vi "TP Editor-Save.vi"(5 "File Name":string, 8 "path":path) -> (0 "error out":errorcluster, 1 "Cancel":bool, 2 "File Name 2":string)   [LabVIEW 2018]
uses:
  Global.vi
panel:
  in  "Cancel":bool
  in  "OK":bool
  in  "Program list":i32(listbox)
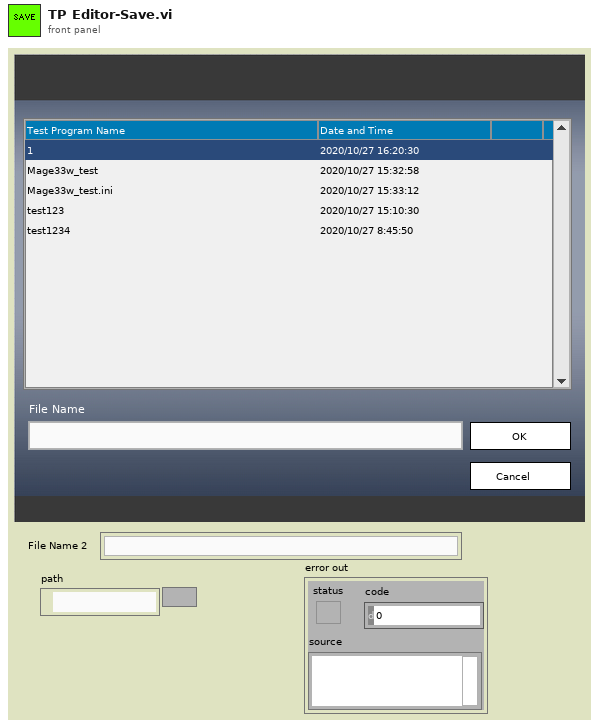
[diagram p1: front panel]
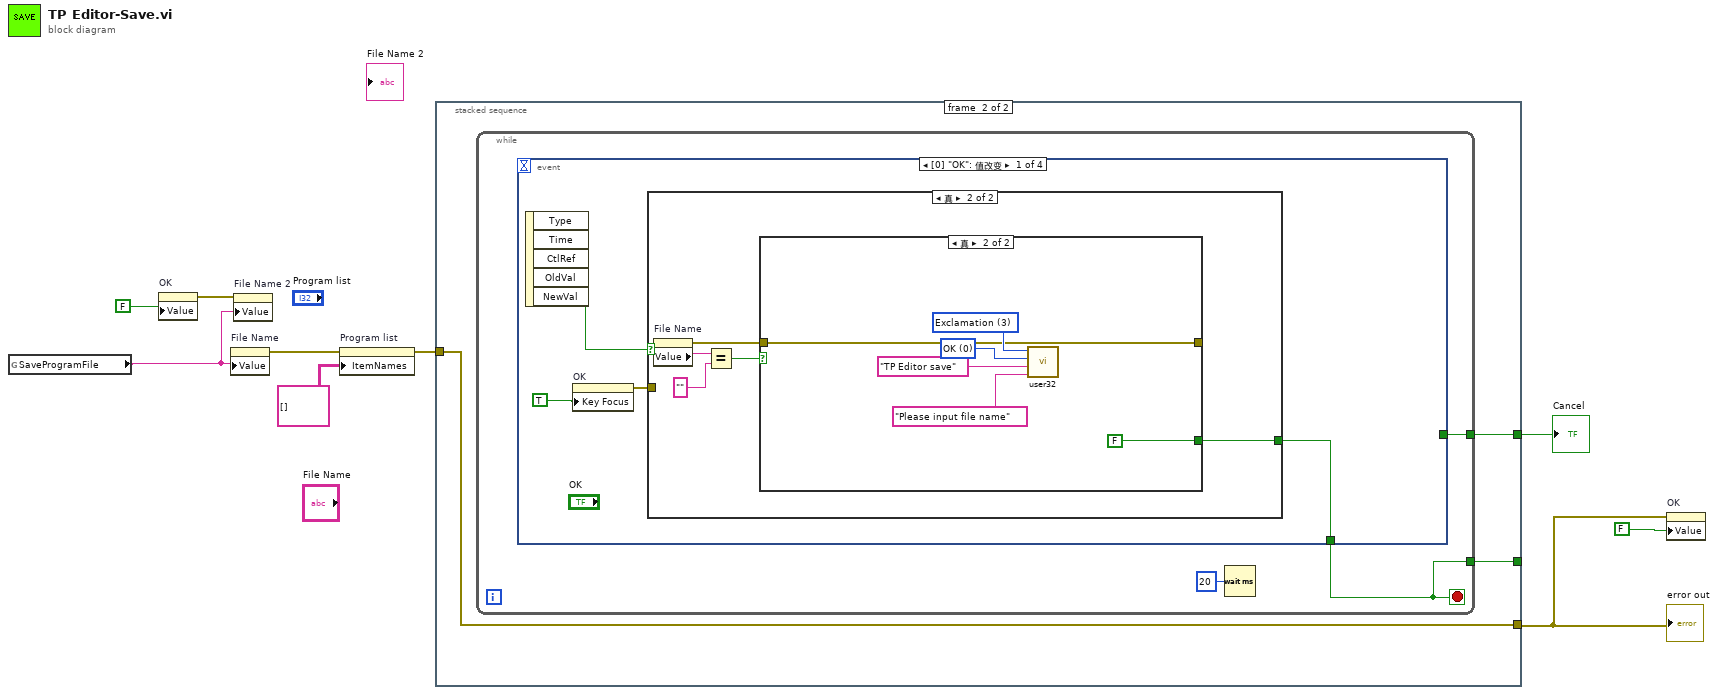
[diagram p0: block diagram]
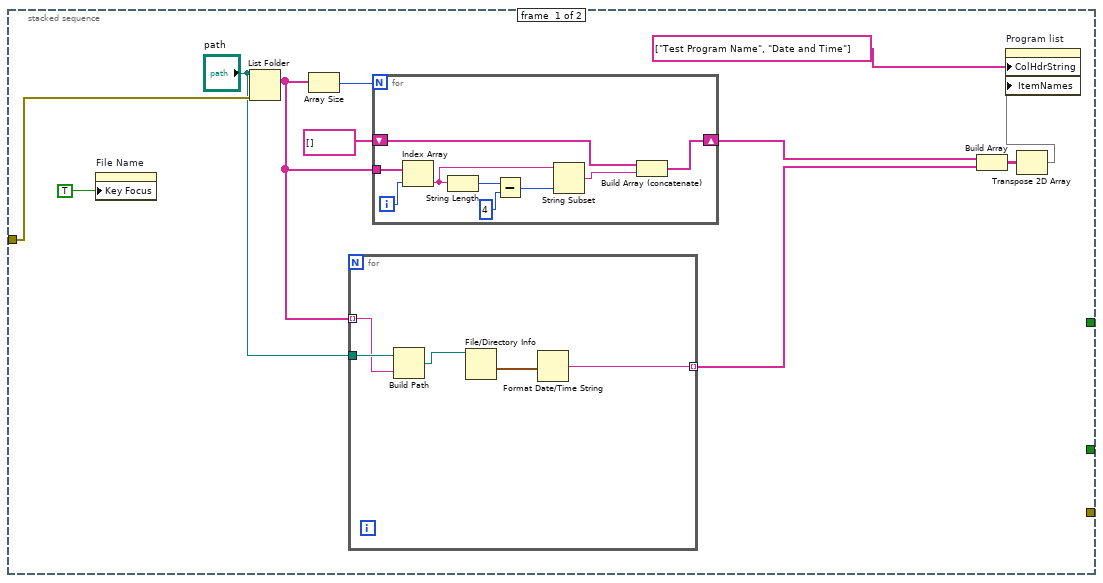
[diagram p2: hidden frame]
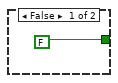
[diagram p3: hidden frame]
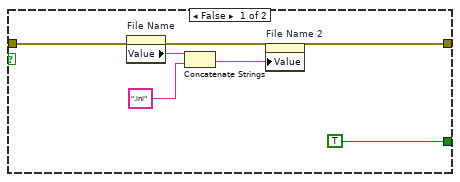
[diagram p4: hidden frame]
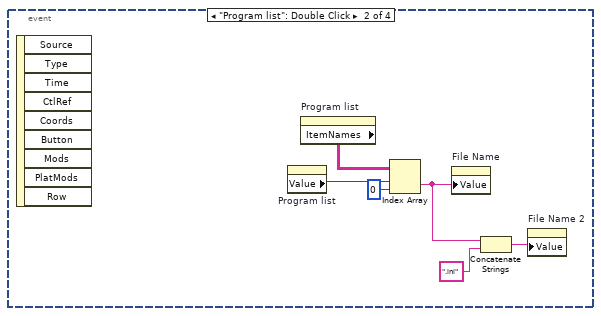
[diagram p5: hidden frame]
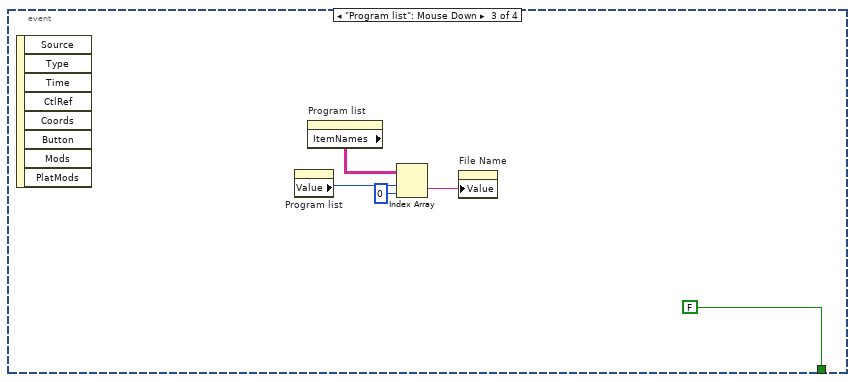
[diagram p6: hidden frame]
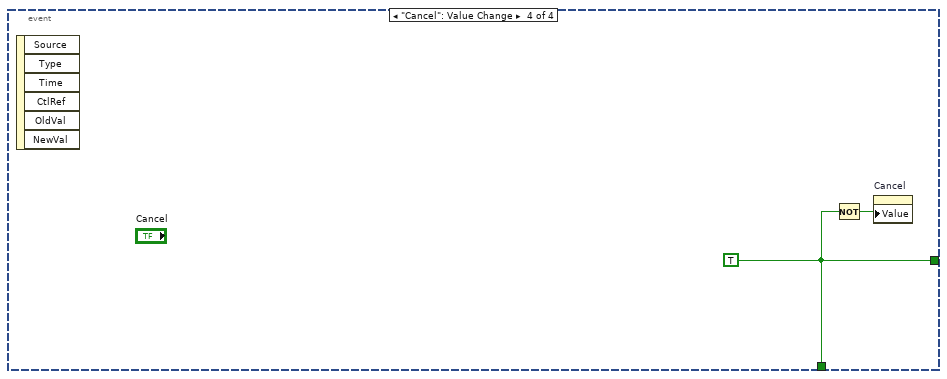
[diagram p7: hidden frame]
diagram:
  n1 = global read "Global.vi" "SaveProgramFile"() -> (w1:string)
  n2 = property on="OK" class="Bool (严格)"("Value"=FALSE) -> (error out=w3:errorcluster)  [unwired: 2 in, 1 out]
  n3 = property on="File Name" class="Str"("Value"=w1) -> (error out=w7:errorcluster)  [unwired: 2 in, 1 out]
  n4 = property on="File Name 2" class="Str"(error in=w3, "Value"=w1) -> ()  [unwired: 1 in, 2 out]
  n5 = property on="Program list" class="MCListbox (严格)"(error in=w7, "ItemNames"=string[][] []) -> (error out=w8:errorcluster)  [unwired: 1 in, 1 out]
  n6 = stacked-sequence {
    tunnel: [_ w37] -> _
    tunnel: w8 -> [w16 w36]
    tunnel: [_ w36] -> w4
    tunnel: [_ w35] -> w6
    frame #0 {
      n7 = property on="File Name" class="Str"("Key Focus"=TRUE) -> ()  [unwired: 2 in, 2 out]
      n8 = List Folder(path="path", error in=w16) -> (filenames=w15:string[])  [unwired: 5 out]
      n9 = Array Size(array=w15) -> (size(s)=w19:i32)
      n10 = for {
        tunnel: w15 -> [w24] mode=indexing
        tunnel: "path" -> [w25]
        tunnel: [w21] -> w11 mode=indexing
        n11 = Build Path(base path=w25, name or relative path=w24) -> (appended path=w23:path)
        n12 = File/Directory Info(path=w23) -> (last mod=w22:timestamp)  [unwired: 1 in, 6 out]
        n13 = Format Date/Time String(seconds (now)=w22) -> (date/time string=w21:string)  [unwired: 2 out]
      }
      n14 = for {
        N: w19 -> [_]
        tunnel: w15 -> [w34]
        shift-right: [w27] -> w10
        shift-left: string[] [] -> [w26]
        i -> [w33]
        n15 = Index Array(array=w34, index=w33) -> (element=w30:string)
        n16 = String Length(string=w30) -> (length=w32:i32)
        n17 = Subtract(x=w32, y=4) -> (x-y=w29:i32)
        n18 = String Subset(string=w30, length (rest)=w29) -> (substring=w28:string)  [unwired: 1 out]
        n19 = Build Array (concatenate)(w26, w28) -> (w27:string[])
      }
      n20 = Build Array(w10, w11) -> (w14:string[][])
      n21 = Transpose 2D Array(2D array=w14) -> (transposed array=w13:string[][])
      n22 = property on="Program list" class="MCListbox (严格)"("ColHdrString"=string[] ["Test Program Name", "Date and Time"] ("Column Header Strings[]"), "ItemNames"=w13) -> ()  [unwired: 2 in, 2 out]
    }
    frame #1 {
      n23 = while {
        tunnel: [w39] -> w37
        tunnel: [w38] -> w35
        stop <- w39 stop-if-true
        n24 = event shown="[0] \"OK\": 值改变" {
          selector: _ -> [_ _ _ _]
          dyn-events: _ -> [_ _ _ _]
          timeout: _ -> [_ _ _ _]
          tunnel: [w44 _ FALSE w73] -> w39
          tunnel: [_ _ _ w73] -> w38
          event "OK": Value Change {
            n25 = event-data() -> ("NewVal"=w43:bool)  [unwired: 5 out]
            n26 = property on="OK" class="Bool (严格)"("Key Focus"=TRUE) -> (error out=w42:errorcluster)  [unwired: 2 in, 1 out]
            n27 = case shown="真" w43 {
              tunnel: [FALSE w47] -> w44
              tunnel: w42 -> [_ _]
              frame False {
              }
              frame True {
                n28 = property on="File Name" class="Str"() -> (error out=w46:errorcluster, "Value"=w50:string)  [unwired: 2 in, 1 out]
                n29 = Equal?(x=w50, y="") -> (x = y?=w48:bool)
                n30 = case shown="真" w48 {
                  tunnel: [TRUE FALSE] -> w47
                  tunnel: w46 -> [w51 w56]
                  tunnel: [w51 w56] -> _
                  frame False {
                    n31 = property on="File Name" class="Str"() -> ("Value"=w55:string)  [unwired: 2 in, 2 out]
                    n32 = Concatenate Strings(w55, ".ini" ("string")) -> (w52:string)
                    n33 = property on="File Name 2" class="Str"("Value"=w52) -> ()  [unwired: 2 in, 2 out]
                  }
                  frame True {
                    w60 = u16 0 items=["OK", "OK+Cancel", "Abort+Retry+Ignore", "Yes+ON+Cancel", "Yes+No", "Retry+Cancel", "Cancel+Retry+Continue"] ("Buttons")
                    w61 = u16 3 items=["None", "Critical", "Question", "Exclamation", "Infomation"] ("Icon")
                    n34 = call "user32.vi"("Icon"=w61, "Buttons"=w60, "Ipcaption"="TP Editor save", "IP Text"="Please input file name") -> ()  [unwired: 2 out]
                  }
                }
              }
            }
          }
          event "Program list": Double Click {
            n35 = event-data() -> ()  [unwired: 10 out]
            n36 = property on="Program list" class="MCListbox (严格)"() -> ("Value"=w66:i32)  [unwired: 2 in, 2 out]
            n37 = property on="Program list" class="MCListbox (严格)"() -> ("ItemNames"=w67:string[][])  [unwired: 2 in, 2 out]
            n38 = Index Array(array=w67, index (row)=w66, index (col)=0 ("disabled index (col)")) -> (element=w63:string)
            n39 = property on="File Name" class="Str"("Value"=w63) -> ()  [unwired: 2 in, 2 out]
            n40 = Concatenate Strings(w63, ".ini" ("string")) -> (w64:string)
            n41 = property on="File Name 2" class="Str"("Value"=w64) -> ()  [unwired: 2 in, 2 out]
          }
          event "Program list": Mouse Down {
            n42 = event-data() -> ()  [unwired: 9 out]
            n43 = property on="Program list" class="MCListbox (严格)"() -> ("Value"=w71:i32)  [unwired: 2 in, 2 out]
            n44 = property on="Program list" class="MCListbox (严格)"() -> ("ItemNames"=w72:string[][])  [unwired: 2 in, 2 out]
            n45 = Index Array(array=w72, index (row)=w71, index (col)=0 ("disabled index (col)")) -> (element=w69:string)
            n46 = property on="File Name" class="Str"("Value"=w69) -> ()  [unwired: 2 in, 2 out]
          }
          event "Cancel": Value Change {
            w73 = TRUE
            n47 = event-data() -> ()  [unwired: 7 out]
            n48 = Not(x=w73) -> (.not. x?=w74:bool)
            n49 = property on="Cancel" class="Bool (严格)"("Value"=w74) -> ()  [unwired: 2 in, 2 out]
          }
        }
        n50 = Wait (ms)(milliseconds to wait=u32 20) -> ()  [unwired: 1 out]
      }
    }
  }
  "error out" <- w4
  "Cancel" <- w6
  n51 = property on="OK" class="Bool (严格)"(error in=w4, "Value"=FALSE) -> ()  [unwired: 1 in, 2 out]
